vi "KLB or Jp2k3D Logging Control Module.vi"() -> ()   [LabVIEW 2012]
doc: "This vi is dynamically run at the start of an acquisition if logging type = jp2000 3D and acquisition mode = experiment. Stop by setting \"Stop?\" via vi server to True.\n\nThis vi continuously checks the JP2000 3D Images to log Buffer FG for \"Completed stack?\" = T; if found the completed stack is removed from the FG and passed to a PCITools VI to compress and then write the stack."
uses:
  PICTools/VIs/Error ring typedef.ctl
  JP2000 3D control/Jp2k 3D image file sets controller mode enum.ctl
  Error Handler/Non-announced error tracker modes enum.ctl
  subvi/KLB globals.vi
  Dynamic Parallel Logging/Parallel image logger globals.vi
  PICTools/VIs/PIC Tools.lvlib
  KLB.lvlib
panel:
  out "elapsed (ms)":u32
  out "# sets processed":i32
  out "last error=T":errorcluster
  out "Error Ring":T1 items=["ERR_NONE"=0, "ERR_EOF"=1, "ERR_SCAN_NON_EXIST"=2, "ERR_REQ_SCAN_NOT_IN_BUF"=3, "ERR_JUNK_BYTES_IN_HEADER"=4, "ERR_JUNK_BYTES_BEFORE_RESTART"=5, "ERR_RESTART_ATTEMPT_AFTER_BAD_DATA"=6, "ERR_TIFF_G34_PASTWIDTH_WARNING"=7, "ERR_MAXOUTPUTSIZE_TOO_SMALL"=8, "ERR_EXTRA_IMAGE_DATA"=9, "ERR_GIF_NO_MORE_PASSES"=10, "ERR_INSUFFICIENT_DATA_FOR_IPTC"=11, "ERR_WHILE_PARSING_IPTC"=12, "ERR_INTERNAL_WATCHDOG"=13, "ERR_NO_PIC_RESOURCE"=-1000, "ERR_BAD_DIB_SIZE"=-1001, "ERR_BAD_NUM_COLORS"=-1002, "ERR_BAD_NUM_GRAYS"=-1003, "ERR_CONFLICTING_REQUEST"=-1004, "ERR_BAD_SEEK"=-1005, "ERR_BAD_READ"=-1006, "ERR_OUT_OF_SPACE"=-1007, "ERR_BAD_DATA"=-1008, "ERR_BAD_IMAGE_TYPE"=-1009, "ERR_BAD_JPEG_DIB_HEADER"=-1010, "ERR_EXPAND_INTERNAL_ERR"=-1011, "ERR_SETUP_NOT_RUN"=-1012, "ERR_UNEXPECTED_EOF"=-1013, "ERR_BAD_WRITE"=-1014, "ERR_BAD_JPEG_COMPONENTS"=-1015, "ERR_UNIMPLEMENTED_FEATURE"=-1016, "ERR_BAD_SUBSAMPLING"=-1017, "ERR_TOO_MANY_INSTANCES"=-1018, "ERR_BAD_INSTANCE_ID"=-1019, "ERR_BAD_WIDTH_OR_HEIGHT"=-1020, "ERR_NOT_ENOUGH_BUFF_SPACE"=-1021, "ERR_BAD_DIB_DIM"=-1022, "ERR_BAD_QUANTIZATION_VALUE"=-1024, "ERR_OUT_OF_DATA"=-1025, "ERR_INCOMPATIBLE_JOIN"=-1026, "ERR_BAD_YUV_OUTPUT_TYPE"=-1027, "ERR_BAD_REGION_INFO"=-1028, "ERR_BAD_COLOR_TRANS_VAL"=-1029, "ERR_BAD_THUMBNAILLEN"=-1030, "ERR_BAD_THUMBNAILTOMAKE"=-1031, "ERR_THUMBNAIL_TOO_BIG"=-1032, "ERR_MISSING_THUMBNAIL"=-1033, "ERR_BAD_PIC2LIST"=-1034, "ERR_BAD_ENDIAN"=-1035, "ERR_CONFLICTING_PIC2LIST_PACKET"=-1036, "ERR_BAD_COLOR_TRANSFORM"=-1037, "ERR_UNSUPPORTED_NUM_COMPONENTS"=-1038, "ERR_STRIPSIZE_TOO_SMALL"=-1039, "ERR_STRIDE_TOO_SMALL"=-1040, "ERR_BAD_PLANAROFFSET"=-1041, "ERR_NOT_BASELINE"=-1101, "ERR_MARKER_ORDER"=-1102, "ERR_FRAME_HEADER"=-1103, "ERR_FILE_OR_FILE_READ"=-1104, "ERR_SCAN_HEADER"=-1105, "ERR_DNL_MARKER"=-1106, "ERR_NUM_LINES"=-1107, "ERR_RESTART"=-1108, "ERR_DC_RESTART"=-1109, "ERR_DECODE_DQ"=-1110, "ERR_DECODE"=-1111, "ERR_SKIP_DC"=-1112, "ERR_DECODE_THUMB"=-1113, "ERR_DECODE_MCU"=-1114, "ERR_SKIP_BLOCK"=-1115, "ERR_RENORM"=-1116, "ERR_AC_RESTART"=-1117, "ERR_DECODE_AC"=-1118, "ERR_DECODE_DC"=-1119, "ERR_BAD_BIT_COUNT"=-1201, "ERR_IMAGE_TOO_WIDE"=-1202, "ERR_MISSING_COLOR_MAP"=-1203, "ERR_BAD_REQUEST"=-1301, "ERR_EXPAND_BAD_SYNCH"=-1302, "ERR_BAD_ZOOM_DIB_HEADERS"=-1401, "ERR_BAD_DES_RECT"=-1402, "ERR_ZOOM_OUT_OF_RANGE"=-1403, "ERR_SRC_REC_TOO_BIG"=-1404, "ERR_DES_REC_TOO_BIG"=-1405, "ERR_BAD_SRC_REC_POS"=-1406, "ERR_BAD_DES_REC_POS"=-1407, "ERR_OUT_OF_ROOM"=-1408, "ERR_BAD_SRC_BITCOUNT"=-1409, "ERR_BAD_DES_BITCOUNT"=-1410, "ERR_COMPRESSED_IMAGE"=-1411, "ERR_BAD_SRC_PALETTE"=-1412, "ERR_BAD_DES_PALETTE"=-1413, "ERR_DES_DIB_TOO_SMALL"=-1414, "ERR_BAD_PIXELBITS"=-1415, "ERR_DIMENSIONS_DISAGREE"=-1416, "ERR_BAD_PIXELTYPES"=-1417, "ERR_BAD_PALETTE"=-1418, "ERR_OPERATION_NOT_INIT"=-1501, "ERR_OPERATION_ALREADY_INIT"=-1502, "ERR_WRONG_MODEL"=-1503, "ERR_UNKNOWN_REQUEST"=-1504, "ERR_UNKNOWN_RESPONSE"=-1505, "ERR_INVALID_OPERATION"=-1506, "ERR_INVALID_VERSION"=-1507, "ERR_GIVEN_BUFF_TOO_SMALL"=-1508, "ERR_APP_BUFF_NULL"=-1509, "ERR_COMMENT_BUFF_NULL"=-1510, "ERR_INVALID_USER_COLORS"=-1511, "ERR_CANT_CREATE_FULL_YUV_BUFF"=-1512, "ERR_NO_VALID_COLORS_AVAIL"=-1513, "ERR_GET_BUFF_INADEQUATE_PADDING"=-1514, "ERR_GET_BUFF_ERR"=-1515, "ERR_PUT_BUFF_ERR"=-1516, "ERR_NOT_8BIT_PRECISION"=-1517, "ERR_NOT_PROGRESSIVE"=-1518, "ERR_MISSING_KEY"=-1519, "ERR_INVALID_KEY"=-1520, "ERR_MAX_NUM_SCANS_EXCEEDED"=-1521, "ERR_UNSUPPORTED_JPEG_FORMAT"=-1522, "ERR_PUT_QUEUE_TOO_SMALL"=-1523, "ERR_TOO_MANY_RESTARTS"=-1524, "ERR_IMAGE_TOO_BIG"=-1525, "ERR_PUT_BUFF_TOO_SMALL"=-1526, "ERR_GET_QUEUE_TOO_SMALL"=-1527, "ERR_BAD_RESTART_INDEX"=-1528, "ERR_INVALID_LAYER"=-1529, "ERR_BAD_EOF"=-1530, "ERR_WRONG_PICL_VERSION"=-1531, "ERR_BAD_SCAN_PARMS"=-1532, "ERR_FULL_IMAGE_NOT_PRESENT"=-1533, "ERR_BAD_COMPRESSION_METHOD"=-1534, "ERR_BAD_COMPRESSION_ORDER"=-1535, "ERR_BAD_HUFFMAN_TABLE"=-1536, "ERR_BAD_QUANT_TABLE"=-1537, "ERR_NOT_LOSSLESS_JPEG"=-1538, "ERR_LJPEG_BAD_NUM_COMPONENTS"=-1539, "ERR_LJPEG_DOES_NOT_SUBSAMPLE"=-1540, "ERR_LJPEG_DOES_NOT_RESTART"=-1541, "ERR_LJPEG_BAD_DC_TABLE"=-1542, "ERR_LJPEG_TOO_MANY_HUFF_TABLES"=-1543, "ERR_LJPEG_MISSING_DIMENSIONS"=-1544, "ERR_LJPEG_BAD_PREDICTOR"=-1545, "ERR_LJPEG_BAD_POINT_TRANSFORM"=-1546, "ERR_QREVERSE"=-1547, "ERR_INTERNAL"=-1548, "ERR_BAD_PTUNING_VALUE"=-1549, "ERR_NOT_PIC2_FILE"=-1550, "ERR_BAD_PIC2_FORMAT"=-1551, "ERR_NOT_PCL2_FILE"=-1552, "ERR_BAD_PACKET_LENGTH"=-1553, "ERR_BAD_PCL2_PACKET"=-1554, "ERR_MISSING_PCL2_PACKET"=-1555, "ERR_BAD_PCL2_VERSION"=-1556, "ERR_BAD_MINOR_VERSION"=-1557, "ERR_TOO_MANY_BITS"=-1558, "ERR_LJPEG_INSUFFICIENT_SRC_ROOM"=-1559, "ERR_LJPEG_PUT_BUFF_TOO_SMALL"=-1560, "ERR_BITERR_MUST_BE_ZERO"=-1561, "ERR_LJPEG_RESTART_ERROR"=-1562, "ERR_LJPEG_BAD_ABE"=-1563, "ERR_LJPEG_BAD_AHT"=-1564, "ERR_IMPROPER_AHT_FOR_IMAGE"=-1565, "ERR_LJPEG_COLOR_NOT_24_BIT"=-1566, "ERR_LJPEG_BAD_MARKER_ORDER"=-1567, "ERR_LJPEG_R_G_OR_B_NOT_8_BITS"=-1568, "ERR_LJPEG_UNSUPPORTED_FILE_TYPE"=-1569, "ERR_BAD_REGION_TYPE"=-1570, "ERR_LJPEG_BAD_BIT_DEPTH"=-1571, "ERR_BAD_PARAMETER_VALUE"=-1572, "ERR_BAD_PRECISIONUCT"=-1573, "ERR_IPTC_TOO_LARGE_FOR_APPD"=-1574, "ERR_NOT_PROTECTED"=-1600, "ERR_BUFF_TOO_SMALL"=-1601, "ERR_WAVELET_INIT"=-1700, "ERR_WAVELET_COMPRESS"=-1701, "ERR_WAVELET_DECOMPRESS"=-1702, "ERR_BAD_IMAGENUMBER"=-1703, "ERR_CHUNKSIZE_TOO_SMALL"=-1704, "ERR_EXTRA_TABLE_OF_RECURSIVE"=-1705, "ERR_SHORT_TABLE_OF_RECURSIVE"=-1706, "ERR_MISSING_TABLE_OF_CLUSTERS"=-1707, "ERR_BAD_TRANSFORMFILTER"=-1708, "ERR_PNG_BAD_HEADER"=-1801, "ERR_PNG_BAD_SIGNATURE"=-1802, "ERR_PNG_MISSING_IHDR"=-1803, "ERR_PNG_BAD_IHDR"=-1804, "ERR_PNG_UNSUPPORTED_FEATURE"=-1805, "ERR_PNG_BAD_BIT_DEPTH"=-1806, "ERR_PNG_UNSUPPORTED_BIT_DEPTH"=-1807, "ERR_PNG_BAD_COLOR_TYPE"=-1808, "ERR_PNG_BAD_PLTE"=-1809, "ERR_PNG_MISSING_IDAT"=-1810, "ERR_PNG_BAD_CHUNK_TYPE"=-1811, "ERR_PNG_MISSING_PLTE"=-1812, "ERR_PNG_BAD_VERSION"=-1813, "ERR_PNG_INTERNAL_ERROR"=-1814, "ERR_PNG_STREAM_ERROR"=-1815, "ERR_PNG_INSUFFICIENT_DATA"=-1816, "ERR_PNG_BAD_CRC"=-1817, "ERR_PNG_BAD_CHUNK_ORDER"=-1818, "ERR_PNG_BAD_COMPRESSION"=-1819, "ERR_PNG_INVALID_FORMAT"=-1820, "ERR_INVALID_BACKGROUND"=-1821, "ERR_INVALID_TRANSPARENCY"=-1822, "ERR_WSQ_MISSING_MARKER"=-1901, "ERR_WSQ_MISSING_SOI"=-1902, "ERR_WSQ_MISSING_DIMENSIONS"=-1903, "ERR_WSQ_BAD_NUM_SUBBANDS"=-1904, "ERR_WSQ_BAD_HUFFMAN_TABLE_LEN"=-1905, "ERR_WSQ_MORE_THAN_8_HUFF_TABLES"=-1906, "ERR_WSQ_BAD_RESTART_HEADER"=-1907, "ERR_WSQ_BAD_FRAME_HEADER"=-1908, "ERR_WSQ_MISSING_SOB_MARKER"=-1909, "ERR_WSQ_UNEXPECTED_MARKER"=-1910, "ERR_WSQ_BAD_BLOCK_HEADER"=-1911, "ERR_WSQ_UNDEFINED_HUFFMAN_TABLE"=-1912, "ERR_WSQ_BAD_DTT_FILTERS"=-1913, "ERR_WSQ_MISSING_ANALYSIS_FILTER"=-1914, "ERR_WSQ_MISSING_SYNTHESIS_FILTER"=-1915, "ERR_WSQ_TOO_FEW_ECS_BLOCKS"=-1916, "ERR_WSQ_MISSING_FRAME_HEADER"=-1917, "ERR_WSQ_BAD_LOGFILE"=-1918, "ERR_WSQ_NO_ACTIVE_SUBBANDS"=-1919, "ERR_UNSUPPORTED_PLATFORM"=-1920, "ERR_NO_STATUS"=-2000, "ERR_USER_ABORTED"=-2001, "ERR_INTERNAL_INVALID_SREQUEST"=-2002, "ERR_HANDLE_NOT_FOUND"=-2003, "ERR_MEMORY_ALLOCATION_ERROR"=-2004, "ERR_FILE_OPEN_ERROR"=-2005, "ERR_DUPLICATE_ID"=-2006, "ERR_INVALID_HANDLE"=-2007, "ERR_LSEEK_ERROR"=-2008, "ERR_MORE"=-2009, "ERR_INTERNAL_POSTMESSAGE"=-2010, "ERR_LOCATE_SERVER_ERROR"=-2011, "ERR_INTERNAL_EXTRA_RESPONSE"=-2012, "ERR_INTERNAL_NOT_IN_PICLIST"=-2013, "ERR_INTERNAL_SHAREDINIT"=-2014, "ERR_INTERNAL_RESPONSE_SIZE"=-2015, "ERR_SERVER_RESPONSE_TIMEOUT"=-2016, "ERR_SERVER_MEMORY_ALLOCATION"=-2017, "ERR_SERVER_REQUEST_SIZE"=-2018, "ERR_SERVER_CLOSE"=-2019, "ERR_PUT_QUEUE_NULL"=-2020, "ERR_ALREADY_IN_PICLIST"=-2021, "ERR_INTERNAL_DELETE_RESPONSE"=-2022, "ERR_TOO_MANY_OPCODES_LOADED"=-2100, "ERR_OPCODE_DLL_NOT_FOUND"=-2101, "ERR_OPCODE_DLL_INVALID"=-2102, "ERR_OPCODE_INTERNAL_ERROR"=-2103, "ERR_OPCODE_INVALID_REG_CODE"=-2104, "ERR_OPCODE_UNSUPPORTED_PARMVER"=-2105, "ERR_LIB_NOT_INIT"=-2106, "ERR_CREATE_THREAD_ERROR"=-2107, "ERR_THREAD_EXITED"=-2108, "ERR_MEM_CHECK"=-2109, "ERR_CALLED_FROM_WRONG_THREAD"=-2110, "ERR_CALLED_FROM_WRONG_FIBER"=-2111, "ERR_DEFER_FROM_WRONG_THREAD"=-2112, "ERR_CREATE_MUTEX_ERROR"=-2113, "ERR_THREAD_ERROR"=-2114, "ERR_MUTEX_ERROR"=-2115, "ERR_EXTRASIZE_ZERO"=-2116, "ERR_DJVU_DECODE_ERR"=-2200, "ERR_DJVU_RENDER_ERR"=-2201, "ERR_DJVU_ENCODE_ERR"=-2202, "ERR_DJVU_MASK_ERR"=-2203, "ERR_DJVU_BADTEXTQUALITY"=-2204, "ERR_NULL_DEFERFN"=-2205, "ERR_DEFERFN_ABORT"=-2206, "ERR_DEFERFN_REQ_CONT"=-2207, "ERR_DEFERFN_16BIT_UNSUPPORTED"=-2208, "ERR_DEFERFN_NEST_PEGASUS"=-2209, "ERR_MODCA_BASE"=-2300, "ERR_MODCA_INVALID_SFI"=-2301, "ERR_MODCA_UNRECOGNIZED_ID"=-2302, "ERR_MODCA_EOD"=-2303, "ERR_IOCA_NOTBILEVEL"=-2304, "ERR_IOCA_EOD"=-2305, "ERR_IOCA_UNSUPPORTED"=-2306, "ERR_IOCA_INVALID"=-2307, "ERR_IOCA_BAD_WIDTH"=-2308, "ERR_CALS_BAD_HEADER"=-2309, "ERR_CALS_NO_WIDTH"=-2310, "ERR_CALS_UNSUPPORTED"=-2311, "ERR_CALS_BAD_RORIENT"=-2312, "ERR_BAD_WIDTHPAD"=-2313, "ERR_MODCA_INVALID_STRUCTURED_FIELD_IDENTIFIER"=-2314, "ERR_MODCA_UNRECOGNIZED_IDENTIFIER_CODE"=-2315, "ERR_MODCA_DATA_STREAM_STATE_VIOLATION"=-2316, "ERR_MODCA_UNRECOGNIZED_STRUCTURED_FIELD_OR_TRIPLET"=-2317, "ERR_MODCA_REQUIRED_STRUCTURED_FIELD_MISSING"=-2318, "ERR_MODCA_REQUIRED_PARAMETER_MISSING"=-2319, "ERR_MODCA_UNACCEPTABLE_PARAMETER_VALUE"=-2320, "ERR_MODCA_INCONSISTENT_PARAMETER_VALUES"=-2321, "ERR_MODCA_UNSUPPORTED"=-2322, "ERR_MODCA_UNABLE_TO_PARSE_PTOCA_FUNCTION"=-2323, "ERR_MODCA_WINDOWS_API_FAILED"=-2324, "ERR_MODCA_CANNOT_FIND_OVERLAY"=-2325, "ERR_MODCA_EXTERNAL_OVERLAY_IS_NULL"=-2326, "ERR_BAD_STATESTAMP"=-2400, "ERR_BAD_RCVRSTATE"=-2401, "ERR_BAD_ROI"=-2402, "ERR_RCVRSTATE_GET_MISMATCH"=-2403, "ERR_BAD_OUTPUTSIZE"=-2404, "ERR_BAD_CRC"=-2405, "ERR_IDP_VERSION_MISMATCH"=-2406, "ERR_BAD_SIGNATURE"=-2407, "ERR_NOT_JPEG_2000"=-2500, "ERR_BAD_MARKER"=-2501, "ERR_BAD_NUM_COMPONENTS"=-2503, "ERR_BAD_MARKER_ORDER"=-2504, "ERR_BAD_BIT_DEPTH"=-2509, "ERR_COLOR_NOT_24_BIT"=-2510, "ERR_BAD_NUM_TILES"=-2516, "ERR_COLOR_MAP_TO_RGB_NOT_8_BIT"=-2517, "ERR_BAD_PALETTE_INFO"=-2518, "ERR_BAD_COMPONENT_MAP_INFO"=-2519, "ERR_UNSUPPORTED_PIXEL_TYPE"=-2520, "ERR_OTHER_PARTITION_NOT_GRAY"=-2521, "ERR_TCT_WAVELET_TRANSFORMS_DIFFER"=-2522, "ERR_BAD_CHANNEL_TRANSFORMATION"=-2524, "ERR_BAD_TILE_DIMENSIONS"=-2526, "ERR_BAD_NUM_PARTITIONS"=-2527, "ERR_OUT_OF_SPACE_FOR_COMPONENT"=-2528, "ERR_INTERNAL_ERR"=-2530, "ERR_PUT_BUFFER_TOO_SMALL"=-2531, "ERR_QUEUE_MAY_NOT_BE_REVERSED"=-2532, "ERR_BAD_STRIDE"=-2534, "ERR_NULL_REGION"=-2535, "ERR_BAD_COMPRESSION_PROFILE"=-2536, "ERR_BAD_DECOMP_OR_SKIPPED_LEVELS"=-2537, "ERR_BAD_NUM_LAYERS"=-2538, "ERR_BAD_PROGRESSION_ORDER"=-2539, "ERR_BAD_TILE_COMP_TRANSFORM"=-2541, "ERR_BAD_WAVELET_TRANSFORM"=-2542, "ERR_BAD_IMAGE_WIDTH_OR_HEIGHT"=-2543, "ERR_BAD_TILE_WIDTH_OR_HEIGHT"=-2544, "ERR_BAD_TILE_OFFSET"=-2545, "ERR_BAD_TILE_ORIENTATION"=-2546, "ERR_COLORMAP_CAN_NOT_BE_SIGNED"=-2547, "ERR_BAD_CROP_PARAMETER"=-2548, "ERR_OFFSET_TOO_BIG"=-2549, "ERR_SIGNED_PIXELS_MAKING_BMP"=-2550, "ERR_BAD_BIT_DEPTH_MAKING_BMP"=-2551, "ERR_INSUFFICIENT_PARTITIONS"=-2552, "ERR_ONLY_2_TO_1_UPSAMPLING"=-2553, "ERR_SUBSAMPLED_CROP_UNSUPPORTED"=-2554, "ERR_UNSUPPORTED_COLOR_MAP_OPTION"=-2555, "ERR_CROP_AREA_EXCEEDS_IMAGE"=-2556, "ERR_PIC2LIST_HAS_DESCRIPTION"=-2557, "ERR_TOO_MANY_TILE_PARTS"=-2558, "ERR_BAD_PRECINCT_WIDTH_OR_HEIGHT"=-2559, "ERR_BAD_PSNR"=-2560, "ERR_BAD_RATE"=-2561, "ERR_BAD_LAYERRATE"=-2562, "ERR_BAD_COMPFILESIZE"=-2563, "ERR_UNSUPPORTED_BMP_IO"=-2564, "ERR_PARTITION_MISMATCH"=-2565, "ERR_UNSUPPORTED_SLICE_ENCODING"=-2566, "ERR_BAD_SLICE_OFFSET"=-2567, "ERR_UPDATEDTILES_NOT_ALLOWED"=-2568, "ERR_J2KLIB_WARNING"=-2569, "ERR_MODE_REQUIRES_SEEKING_ENABLED"=-2570, "ERR_BAD_SCAN_NUM"=-2601, "ERR_UNSUPPORTED_COMPONENT_DIMENSIONS"=-2602, "ERR_BAD_RESTART_INTERVAL"=-2605, "ERR_MISSING_DIMENSIONS"=-2608, "ERR_BAD_SYNCH_AT_EOS"=-2615, "ERR_MISSING_SOS"=-2616, "ERR_BAD_MAXVAL"=-2617, "ERR_BAD_RESET"=-2618, "ERR_BAD_NEARPARAM"=-2619, "ERR_BAD_ILVPARAM"=-2620, "ERR_BAD_PT"=-2621, "ERR_PTWITHMAP"=-2622, "ERR_BAD_MARKER_LENGTH"=-2623, "ERR_UNEXPECTED_UNKNOWN_LENGTH"=-2700, "ERR_UNSUPPORTED_UNPACKED_PIXELS"=-2701, "ERR_ENCODEMODE_LOSSY_TEXT_NOT_LOSSLESS"=-2702, "ERR_ENCODEMODE_LOSSY_HALFTONE_NOT_LOSSLESS"=-2703, "ERR_UNSUPPORTED_SEGMENT_REFERENCES"=-2704, "ERR_PCD_UNKNOWN_ERROR"=-3000, "ERR_PCD_BAD_FORMAT"=-3001, "ERR_PCD_BAD_PARAMETER"=-3002, "ERR_PCD_BAD_VERSION"=-3003, "ERR_PCD_READ_ERROR"=-3004, "ERR_PCD_CLOSE_ERROR"=-3005, "ERR_PCD_SEEK_ERROR"=-3006, "ERR_PCD_OPEN_ERROR"=-3007, "ERR_PCD_BAD_KEY"=-3008, "ERR_PCD_KEY_REQUIRED"=-3009, "ERR_PCD_ENCRYPTION_ERROR"=-3010, "ERR_PCD_NOT_INTERLEAVED"=-3011, "ERR_PCD_UNKNOWN_ATTRIBUTE"=-3012, "ERR_PCD_MEMORY_ERROR"=-3013, "ERR_PCD_SIZE_NOT_FOUND"=-3014, "ERR_OBJECT_INSTANCE_CORRUPT"=-3100, "ERR_BAD_X_VALUE"=-3101, "ERR_BAD_Y_VALUE"=-3102, "ERR_BAD_ARRAY_INDEX"=-3103, "ERR_BAD_RESOLUTION"=-3104, "ERR_BAD_DETECTION_QUALITY"=-3105, "ERR_BAD_SPECK_WIDTH"=-3106, "ERR_BAD_SPECK_HEIGHT"=-3107, "ERR_BAD_HORZ_LINE_MIN_LENGTH"=-3108, "ERR_BAD_HORZ_LINE_MAX_THICKNESS"=-3109, "ERR_BAD_HORZ_LINE_MIN_ASPECT_RATIO"=-3110, "ERR_BAD_HORZ_LINE_MAX_GAP"=-3111, "ERR_BAD_HORZ_LINE_MAX_CHAR_REPAIR_SIZE"=-3112, "ERR_BAD_HORZ_LINE_EDGE_CLEANING"=-3113, "ERR_BAD_VERT_LINE_MIN_LENGTH"=-3114, "ERR_BAD_VERT_LINE_MAX_THICKNESS"=-3115, "ERR_BAD_VERT_LINE_MIN_ASPECT_RATIO"=-3116, "ERR_BAD_VERT_LINE_MAX_GAP"=-3117, "ERR_BAD_VERT_LINE_MAX_CHAR_REPAIR_SIZE"=-3118, "ERR_BAD_VERT_LINE_EDGE_CLEANING"=-3119, "ERR_BAD_HORZ_ROTATION_ANGLE"=-3120, "ERR_BAD_VERT_ROTATION_ANGLE"=-3121, "ERR_BAD_SHEAR_ANGLE"=-3122, "ERR_BAD_AMOUNT_OF_EFFECT_LEFT"=-3123, "ERR_BAD_AMOUNT_OF_EFFECT_RIGHT"=-3124, "ERR_BAD_AMOUNT_OF_EFFECT_UP"=-3125, "ERR_BAD_AMOUNT_OF_EFFECT_DOWN"=-3126, "ERR_BAD_DIAGONAL_DIRECTION"=-3127, "ERR_BAD_RECT_WIDTH"=-3128, "ERR_BAD_RECT_HEIGHT"=-3129, "ERR_BAD_PAD_COLOR"=-3130, "ERR_BAD_MIN_DENSITY"=-3131, "ERR_BAD_MIN_PIXEL_COUNT"=-3132, "ERR_BAD_MAX_PIXEL_COUNT"=-3133, "ERR_BAD_HORIZONTAL_MAGNIFICATION"=-3134, "ERR_BAD_VERTICAL_MAGNIFICATION"=-3135, "ERR_BAD_MINIMUM_AREA_WIDTH"=-3136, "ERR_BAD_MINIMUM_AREA_HEIGHT"=-3137, "ERR_BAD_VERTICAL_SIZE_ADJUSTMENT"=-3138, "ERR_BAD_HORIZONTAL_SIZE_ADJUSTMENT"=-3139, "ERR_BAD_DENSITY"=-3140, "ERR_BAD_MAXIMUM_DOT_SIZE"=-3141, "ERR_BAD_VERIFICATION_HEIGHT"=-3142, "ERR_BAD_MINIMUM_BLACK_ON_EDGES"=-3143, "ERR_BAD_AMOUNT"=-3144, "ERR_IMAGE_TOO_SMALL"=-3145, "ERR_BAD_BORDER_SPECK_SIZE"=-3146, "ERR_BAD_PAGE_SPECK_SIZE"=-3147, "ERR_BAD_MINIMUM_PAGE_WIDTH"=-3148, "ERR_BAD_MAXIMUM_PAGE_WIDTH"=-3149, "ERR_BAD_MINIMUM_PAGE_HEIGHT"=-3150, "ERR_BAD_MAXIMUM_PAGE_HEIGHT"=-3151, "ERR_BAD_AMOUNT_TO_EXPAND_PAGE"=-3152, "ERR_BAD_HORZ_REG_RESULTANT_MARGIN"=-3153, "ERR_BAD_HORZ_REG_SKIP_DISTANCE"=-3154, "ERR_BAD_HORZ_REG_MIN_BACKGROUND"=-3155, "ERR_BAD_HORZ_REG_MIN_FOREGROUND"=-3156, "ERR_BAD_HORZ_REG_MIN_ACTIVITY"=-3157, "ERR_BAD_HORZ_REG_TO_LINE_MIN_LINE_LENGTH"=-3158, "ERR_BAD_HORZ_REG_TO_LINE_MAX_LINE_GAP"=-3159, "ERR_BAD_HORZ_REG_TO_LINE_MAX_LINE_THICKNESS"=-3160, "ERR_BAD_REG_ACTIVE"=-3161, "ERR_BAD_VERT_REG_RESULTANT_MARGIN"=-3163, "ERR_BAD_VERT_REG_SKIP_DISTANCE"=-3164, "ERR_BAD_VERT_REG_MIN_BACKGROUND"=-3165, "ERR_BAD_VERT_REG_MIN_FOREGROUND"=-3166, "ERR_BAD_VERT_REG_MIN_ACTIVITY"=-3167, "ERR_BAD_VERT_REG_TO_LINE_MIN_LINE_LENGTH"=-3168, "ERR_BAD_VERT_REG_TO_LINE_MAX_LINE_GAP"=-3169, "ERR_BAD_VERT_REG_TO_LINE_MAX_LINE_THICKNESS"=-3170, "ERR_BAD_COMB_LENGTH"=-3171, "ERR_BAD_COMB_HEIGHT"=-3172, "ERR_BAD_COMB_SPACING"=-3173, "ERR_BAD_COMB_H_LINE_THICKNESS"=-3174, "ERR_BAD_COMB_V_LINE_THICKNESS"=-3175, "ERR_BAD_COMB_MIN_CONFIDENCE"=-3176, "ERR_BAD_SENSITIVITY"=-3177, "ERR_BAD_MIN_SATURATION"=-3178, "ERR_BAD_MIN_SIZE"=-3179, "ERR_BAD_BOX_OVERLAP"=-3180, "ERR_BAD_COUNT"=-3181, "ERR_BAD_WHITE_BALANCE_METHOD"=-3200, "ERR_BAD_INTERPOLATION_METHOD"=-3201, "ERR_BAD_RED_FACTOR"=-3202, "ERR_BAD_BLUE_FACTOR"=-3203, "ERR_BAD_BRIGHTNESS_FACTOR"=-3204, "ERR_BAD_GAMMA"=-3205, "ERR_BAD_REGION_FLAGS"=-3206, "ERR_THUMBNAILBUFFER_NOT_NULL"=-3207, "ERR_REDEYE_RECT_LIST_TOO_SHORT"=-3300, "ERR_JPIP_BAD_REQUEST"=-3400, "ERR_JPIP_BAD_RESPONSE"=-3401, "ERR_UNKNOWN_ACTION"=-3402, "ERR_CHANNEL_NOT_OPEN"=-3403, "ERR_TOO_MANY_CHANNELS"=-3404, "ERR_TID_NOT_ALLOWED"=-3405, "ERR_TID_MISSING"=-3406, "ERR_CID_NOT_ALLOWED"=-3407, "ERR_CID_MISSING"=-3408, "ERR_UNSUPPORTED_TRANSPORT"=-3409, "ERR_BAD_JPIPREQUESTSTRING"=-3410, "ERR_BAD_JPIPRESPONSESTRING"=-3411, "ERR_BAD_TARGET"=-3412, "ERR_BAD_TARGETID"=-3413, "ERR_BAD_JPIPCHANNELID"=-3414, "ERR_BAD_JPIPCHANNELIDSCLOSE"=-3415, "ERR_BAD_MODEL"=-3416, "ERR_BAD_GRANTEDJPIPCHANNELID"=-3417, "ERR_BAD_GRANTEDJPIPCHANNELHOST"=-3418, "ERR_BAD_GRANTEDJPIPCHANNELPATH"=-3419, "ERR_BAD_EORMESSAGEBODY"=-3420, "ERR_STATELESS_SECOND_REQUEST"=-3421, "ERR_NOT_DEFAULT_MEDIATYPE"=-3422, "ERR_UNSUPPORTED_MEDIATYPE"=-3423, "ERR_NOT_ALLOWED_TRANSPORT"=-3424, "ERR_BAD_TPMODEL"=-3425, "ERR_UNSUPPORTED_JPX_FORMAT"=-3500, "ERR_BAD_JPEG2000PROFILE"=-3501, "ERR_BAD_JPEG2000FILEFORMAT"=-3502, "ERR_BAD_TILECOMPFLAGS"=-3503, "ERR_BAD_THUMBNAIL"=-3504, "ERR_TOO_MANY_DISCARD_LAYERS"=-3505, "ERR_BAD_RESOLUTIONBOX_VALUE"=-3506, "ERR_MISSING_ICC_PROFILE_DATA"=-3507, "ERR_EXIFIFD_CONTEXT"=-3600, "ERR_GPSINFOIFD_CONTEXT"=-3601, "ERR_INTEROPERABILITYIFD_CONTEXT"=-3602, "ERR_LIBRARY_ERROR"=-3603, "ERR_BAD_PIXTYPE"=-3604, "ERR_UNSUPPORTED_PIXELFORMAT"=-3605, "ERR_BAD_OVERLAP"=-3606, "ERR_BAD_TRIMMED_FLEXBITS"=-3607, "ERR_BAD_SUBBANDS"=-3608, "ERR_BAD_ALPHA_CHANNEL_FORMAT"=-3609, "ERR_IMAGE_DATA_MUST_BE_UNCOMPRESSED"=-3610, "ERR_SUBSAMPLING_DISALLOWED_FOR_PIXTYPE"=-3611, "ERR_BAD_REORIENTATION"=-3612, "ERR_UNSUPPORTED_INPUT_IMAGE"=-3613, "JWBASE"=-7000, "ERR_UNEXPECTED_RESPONSE"=-7002, "ERR_OUT_OF_MEMORY"=-7003, "ERR_UNSUPPORTED_FILE_TYPE"=-7004, "ERR_BAD_STRUCTURE_PARAMETER"=-7005, "ERR_INVALID_HEADER_INFO"=-7006, "ERR_BAD_RLE_DATA"=-7007, "ERR_RLE_DELTA_UNSUPPORTED"=-7008, "ERR_BAD_BMP_TYPE"=-7009, "ERR_NULL_POINTER"=-7010, "ERR_BAD_TGA_TYPE"=-7011, "ERR_UNSUPPORTED_BIT_DEPTH"=-7012, "ERR_UNSUPPORTED_RLE_MODE"=-7013, "ERR_BAD_PCX_PALETTE"=-7014, "ERR_NOT_BMP_FILE"=-7015, "ERR_NOT_TARGA_FILE"=-7016, "ERR_NOT_PCX_FILE"=-7017, "ERR_NOT_GIF_FILE"=-7018, "ERR_BAD_GIF_SEPARATOR"=-7019, "ERR_DIFFERENT_GIF_FORMAT"=-7020, "ERR_GIF_DECODE_ERROR_1"=-7021, "ERR_GIF_DECODE_ERROR_2"=-7022, "ERR_GIF_DECODE_ERROR_3"=-7023, "ERR_GIF_DECODE_ERROR_4"=-7024, "ERR_GIF_DECODE_ERROR_5"=-7025, "ERR_GIF_DECODE_ERROR_6"=-7026, "ERR_BAD_GIF_EXTENSION_BLOCK"=-7027, "ERR_NOT_TIFF_FILE"=-7028, "ERR_INVALID_TIFF_IFD_COUNT"=-7029, "ERR_INVALID_TIFF_TAG"=-7030, "ERR_TIFF_NO_JPEG"=-7031, "ERR_TIFF_NO_CCITT"=-7032, "ERR_TIFF_NO_DIFFERENCING"=-7033, "ERR_TIFF_NO_TILES"=-7034, "ERR_TIFF_NO_CMYK"=-7035, "ERR_TIFF_NO_YCbCr"=-7036, "ERR_TIFF_BAD_PHOTOMETRIC"=-7037, "ERR_TIFF_UNSUPPORTED_COMPRESSION"=-7038, "ERR_TIFF_NO_STRIP_INFO"=-7039, "ERR_TIFF_NEED_COLORMAP"=-7040, "ERR_TIFF_PALETTE_WRONG_SIZE"=-7041, "ERR_TIFF_BAD_STRIPOFFSETS_TYPE"=-7042, "ERR_TIFF_NO_WIDTH_OR_LENGTH"=-7043, "ERR_TIFF_TOO_FEW_STRIPS"=-7044, "ERR_TIFF_TAG_COUNT_SHOULD_BE_1"=-7045, "ERR_TIFF_UNEXPECTED_TYPE"=-7046, "ERR_TIFF_BAD_ARRAY_TYPE"=-7047, "ERR_TIFF_BAD_ARRAY_COUNT"=-7048, "ERR_TIFF_BAD_BITS_PER_SAMPLE"=-7049, "ERR_UNKNOWN_UTILITY_FUNCTION"=-7050, "ERR_BAD_OUTPUT_BPP"=-7051, "ERR_BAD_INPUT_PALETTE"=-7052, "ERR_INVALID_NUMBER_OF_OUTPUT_COLORS"=-7053, "ERR_BAD_INPUT_PIXEL_DEPTH"=-7054, "ERR_DIB_MUST_BE_UNCOMPRESSED"=-7055, "ERR_MISSING_PALETTE"=-7056, "ERR_INVALID_STRUCTURE_SIZE"=-7057, "ERR_BAD_PROGRESSIVE_MODE"=-7058, "ERR_NOT_YET_IMPLEMENTED"=-7059, "ERR_BAD_NUMBER_OF_PLANES"=-7060, "ERR_INVALID_TARGA_BPP"=-7061, "ERR_UNSUPPORTED_INPUT_PIXEL_DEPTH"=-7062, "ERR_TIFF_LOGIC_ERROR_1"=-7063, "ERR_TIFF_LOGIC_ERROR_2"=-7064, "ERR_TIFF_OUTPUT_WIDTH_0"=-7065, "ERR_UTL_HISTOGRAM_IS_NULL"=-7066, "ERR_UTL_COLORMAP_IS_NULL"=-7067, "ERR_TOO_MANY_COLORS_IN_COLORMAP"=-7068, "ERR_DIB_MUST_BE_24BPP"=-7069, "ERR_INVALID_HISTOGRAM_SIZE"=-7070, "ERR_UNSUPPORTED_TGA_ATT_BITS"=-7071, "ERR_UNIMPLEMENTED_SUBCODE"=-7072, "ERR_TIFF_UNSUPPORTED_ORIENTATION"=-7073, "ERR_TIFF_NO_SAMPLEFORMAT"=-7074, "ERR_TIFF_UNSUPPORTED_DATATYPE"=-7075, "ERR_SUB8_PTR3_NULL"=-7076, "ERR_PALETTE_SIZE"=-7077, "ERR_COLOR_COUNT_MISMATCH"=-7078, "ERR_BAD_DIB_DEPTH"=-7079, "ERR_UTL_NO_EXTERNAL_PALETTE"=-7080, "ERR_SUB8_LOGIC_ERROR_1"=-7081, "ERR_OUTPUT_QUEUE_TOO_SMALL"=-7082, "ERR_SUBCODE_INTERNAL_1"=-7083, "ERR_SUBCODE_INTERNAL_2"=-7084, "ERR_SUBCODE_INTERNAL_3"=-7085, "ERR_SUBCODE_INTERNAL_4"=-7086, "ERR_SUBCODE_INTERNAL_5"=-7087, "ERR_PCD_NOT_VALID_COMPRESSION"=-7088, "ERR_PCD_NO_NAME"=-7089, "ERR_PCD_BAD_RESOLUTION"=-7090, "ERR_TIFF_G34_1"=-7091, "ERR_TIFF_G34_2"=-7092, "ERR_TIFF_G34_3"=-7093, "ERR_TIFF_G34_4"=-7094, "ERR_TIFF_G34_5"=-7095, "ERR_TIFF_G34_6"=-7096, "ERR_TIFF_G34_7"=-7097, "ERR_TIFF_G34_8"=-7098, "ERR_TIFF_G3_DECODE_1"=-7099, "ERR_TIFF_G3_DECODE_2"=-7100, "ERR_TIFF_G3_DECODE_3"=-7101, "ERR_TIFF_G3_DECODE_4"=-7102, "ERR_TIFF_LZW_DECODE_1"=-7103, "ERR_TIFF_BAD_PREDICTOR"=-7104, "ERR_TIFF_UNSUPPORTED_PLANARCONFIGURATION"=-7105, "ERR_TIFF_UNSUPPORTED_SAMPLES_PER_PIXEL"=-7106, "ERR_QUEUE_ERROR"=-7107, "ERR_TIFF_BAD_FILLORDER"=-7108, "ERR_TIFF_G34_RAWWIDTH0"=-7109, "ERR_TIFF_G34_INVALIDEOL"=-7110, "ERR_TIFF_G34_PASTWIDTH"=-7111, "ERR_TIFF_G34_PREMATUREEOS"=-7112, "ERR_TIFF_G34_FIRSTLINE2D"=-7113, "ERR_TIFF_G34_EXTENSIONCODE"=-7114, "ERR_TIFF_G34_INVALIDCODE"=-7115, "ERR_TIFF_G34_SEQUENCE"=-7116, "ERR_TIFF_G34_G32DMISSINGEOL"=-7117, "ERR_INVALID_BISIZE"=-7118, "ERR_INVALID_CMYK_PARAMETERS"=-7119, "ERR_PUTQ_UNEXPECTED_EOF"=-7120, "ERR_PUTQ_BAD_READ"=-7121, "ERR_PUTQ_GET_BUFF_ERR"=-7122, "ERR_TIFF_INVALID_MULTI_ENDIAN"=-7123, "ERR_TIFF_NO_LOSSLESS_JPEG"=-7124, "ERR_TIFF_JPEG_STRIPS"=-7125, "ERR_TIFF_INVALID_PAGE"=-7126, "ERR_TIFF_DUPLICATE_TAG"=-7127, "ERR_THRESHOLD_EXCEEDED"=-7128, "ERR_BAD_THRESHOLD"=-7129, "ERR_BAD_OFFSET"=-7130, "ERR_BAD_DCX_IMAGE"=-7131, "ERR_OUT_OF_ROOM_IN_DCX_FILE"=-7132, "ERR_BAD_CONTRASTFIXEDPOINT"=-7133, "ERR_ALPHA_UNSUPPORTED_FOR_INPUT"=-7134, "ERR_SAVE_ALPHA_REQUIRES_ALPHA_INPUT"=-7135, "ERR_ALPHA_UNSUPPORTED_FOR_OUTPUT"=-7136, "ERR_MASKBUFFERSIZE_TOO_SMALL"=-7137, "ERR_NO_TILE_OFFSETS"=-7138, "ERR_UNSUPPORTED_TILE_WIDTH"=-7139, "ERR_DAMAGED_FILE"=-7200, "ERR_INVALID_DICT"=-7201, "ERR_INVALID_TYPE"=-7202, "ERR_INVALID_HEADER"=-7203, "ERR_MISSING_RESOURCES"=-7204, "ERR_BLANK_PAGE"=-7205, "ERR_NO_IMAGE_FOUND"=-7206, "ERR_INVALID_IMAGE_BPP"=-7207, "ERR_INVALID_IMAGE_HEIGHT"=-7208, "ERR_INVALID_IMAGE_WIDTH"=-7209, "ERR_INVALID_STREAM_LENGTH"=-7210, "ERR_INVALID_PAGE_NUMBER"=-7211, "ERR_INVALID_DICT_KEY"=-7212, "ERR_DAMAGED_XREF_SECTION"=-7213, "ERR_MAX_ARRAY_SIZE_REACHED"=-7214, "ERR_MAX_DICT_SIZE_REACHED"=-7215, "ERR_MAX_STR_LENGTH_REACHED"=-7216, "ERR_MAX_NAME_LENGTH_REACHED"=-7217, "ERR_INVALID_STREAM"=-7218, "ERR_MULT_DECODE_PARMS_NOT_SUPPORTED"=-7219, "ERR_MULT_FILTERS_NOT_SUPPORTED"=-7220, "ERR_UNEXPECTED_NULL_OBJECT"=-7221, "ERR_MULT_CONTENT_STREAMS_NOT_SUPPORTED"=-7222, "ERR_ENCODED_STREAMS_NOT_SUPPORTED"=-7223, "ERR_COLOR_SPACE_NOT_SUPPORTED"=-7224, "ERR_NO_IMAGE_SCALE_TRANSFORM_FOUND"=-7225, "ERR_XREF_OBJ_FOR_TRAILER_NOT_SUPPORTED"=-7226, "ERR_LAYOUT_DOES_NOT_EXIST"=-7300, "ERR_TRUNCATE64"=-7900, "ERR_J2KLIB_OFFSET"=-8000, "ERR_UNEXPECTED_ERROR"=-9000]
  out "Compression Ratio":dbl=2.0
  in  "Stop?":bool
  out "error out":errorcluster
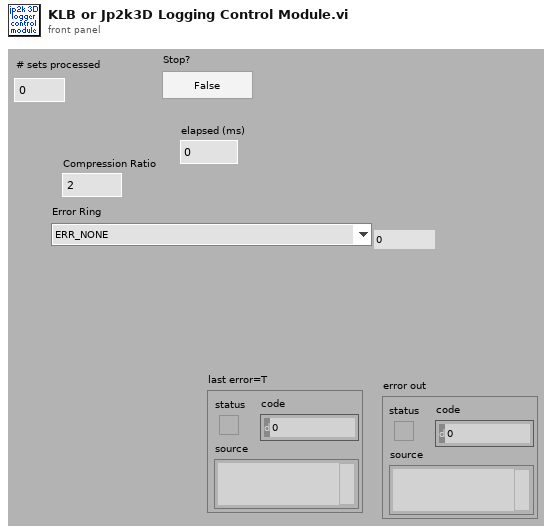
[diagram p1: front panel]
types:
  T1 = typedef "PIC Tools.lvlib/Error ring typedef.ctl" = i32
  T2 = typedef "Jp2k 3D image file sets controller mode enum.ctl" = enum16{"Initialize", "Read registers", "Add Image", "Remove element", "Mark all done 1 camera"}
  T3 = typedef "Non-announced error tracker modes enum.ctl" = enum16{"Reset", "Add error", "Read registers"}
  T4 = typedef "Jp2k file SET cluster.ctl" = cluster{"Path":path, "Camera index":i32, "[Buffer #]":i32[], "Completed?":bool}
  T5 = typedef "IMAQ Image.ctl" = refnum<image>
  T6 = typedef "KLB.lvlib/KLB Settings Cluster.ctl" = cluster{"Logical Cores":T7, "pixelSize (um)":sgl[], "blockSize":u32[], "compressionType":T8, "metadata":string}
  T7 = typedef "KLB.lvlib/KLB # of CPUs enum.ctl" = enum16{"CPU 25%", "CPU 50%", "CPU 75%", "CPU All but 1", "1", "4", "8", "16"}
  T8 = typedef "KLB.lvlib/KLB compression type enum.ctl" = enum8{"Uncompressed", "BZip2"}
  T9 = typedef "PIC Tools.lvlib/Compression options cluster.ctl" = cluster{"Number of Threads":i32, "Lossless compression":bool, "3D compression":bool, "Compression Ratio":dbl}
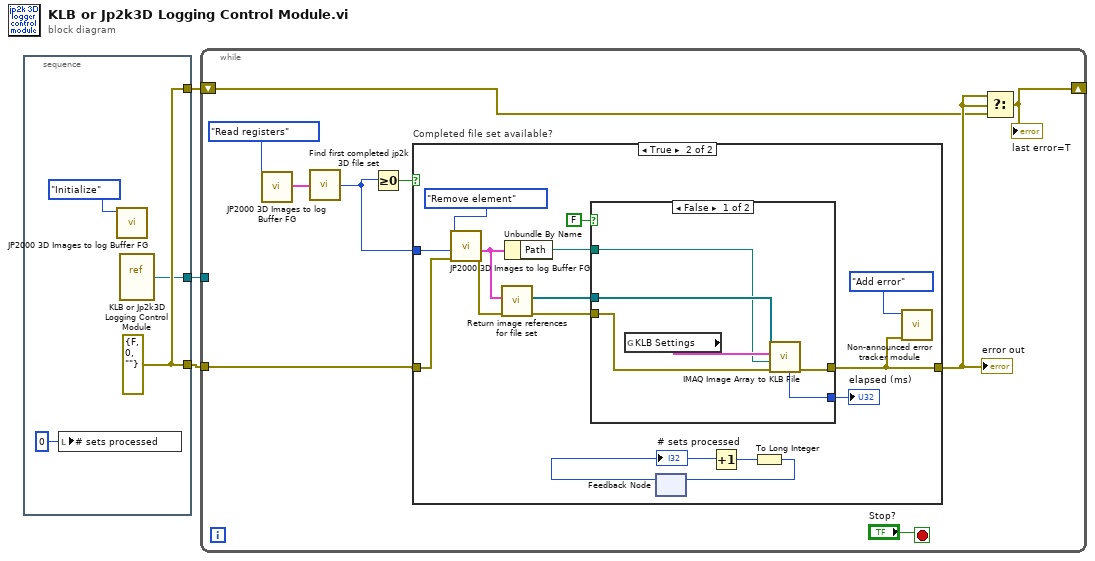
[diagram p0: block diagram]
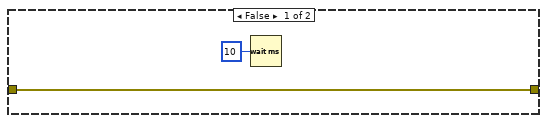
[diagram p2: hidden frame]
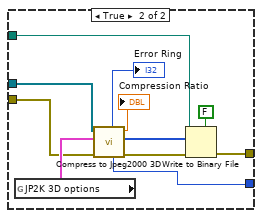
[diagram p3: hidden frame]
diagram:
  n1 = stacked-sequence {
    tunnel: [w6] -> w3
    tunnel: [w6] -> w2
    tunnel: [w5] -> w1
    frame #0 {
      w6 = errorcluster {"status"=FALSE, "code"=0, "source"=""} ("error out")
      n2 = local write "# sets processed"(0 ("# sets processed")) -> ()
      n3 = call "JP2000 3D Images to log Buffer FG.vi"("Mode"=Jp2k_3D_image_file_sets_controller_mode_enum."Initialize") -> ()  [unwired: 8 in, 3 out]
      n4 = vi-ref "KLB or Jp2k3D Logging Control Module.vi"() -> (w5:refnum<vi>)
    }
  }
  n5 = while {
    tunnel: w3 -> [w11]
    shift-right: [w8] -> _
    shift-left: w2 -> [w9]
    tunnel: w1 -> [_]
    stop <- "Stop?" stop-if-true
    n6 = call "JP2000 3D Images to log Buffer FG.vi"("Mode"=Jp2k_3D_image_file_sets_controller_mode_enum."Read registers") -> ("[File sets]"=w13:T4[])  [unwired: 8 in, 2 out]
    n7 = call "Find first completed jp2k 3D file set.vi"("[File sets]"=w13) -> ("1st Completed index"=w12:i32)  [unwired: 4 in]
    n8 = Greater Or Equal To 0?(x=w12) -> (x >= 0?=w15:bool)
    n9 = case "Completed file set available?" shown="True" w15 {
      tunnel: [w18 w21] -> w10
      tunnel: w11 -> [w18 w27]
      tunnel: w12 -> [_ w33]
      frame False {
        n10 = Wait (ms)(milliseconds to wait=u32 10) -> ()  [unwired: 1 out]
      }
      frame True {
        n11 = call "JP2000 3D Images to log Buffer FG.vi"("error in (no error)"=w27, "Index"=w33, "Mode"=Jp2k_3D_image_file_sets_controller_mode_enum."Remove element") -> ("error out"=w26:errorcluster, "Removed element"=w30:T4)  [unwired: 6 in, 1 out]
        n12 = call "Return image references for file set.vi"("error in (no error)"=w26, "Removed element"=w30) -> ("error out"=w29:errorcluster, "Images"=w28:T5[])  [unwired: 8 in]
        n13 = Unbundle By Name(w30) -> ("Path"=w32:path)
        n14 = case shown="False" FALSE {
          tunnel: w32 -> [w36 w46]
          tunnel: w29 -> [w35 w43]
          tunnel: w28 -> [w38 w42]
          tunnel: [w39 w41] -> w21
          tunnel: [w34 w40] -> w19
          frame False {
            n15 = global read "KLB globals.vi" "KLB Settings"() -> (w37:T6)
            n16 = call "IMAQ Image Array to KLB File.vi"("error in (no error)"=w35, "path"=w36, "KLB Settings"=w37, "Images to Compress"=w38) -> ("error out"=w39:errorcluster, "elapsed (ms)"=w34:u32)  [unwired: 6 in]
          }
          frame True {
            n17 = global read "Parallel image logger globals.vi" "JP2K 3D options"() -> (w50:T9)
            n18 = call "Compress to Jpeg2000 3D.vi"("error in"=w43, "Compression options"=w50, "Images to Compress"=w42) -> ("error out"=w48:errorcluster, "OutputBuffer"=w47:u8[], "Compression Ratio achieved"=→"Compression Ratio":dbl, "elapsed (ms)"=w40:u32, "Error Ring"=→"Error Ring":T1)  [unwired: 3 in, 1 out]
            n19 = Write to Binary File(file (use dialog)=w46, data=w47, error in=w48, 5:FALSE ("prepend array or string size? (T)")) -> (error out=w41:errorcluster)  [unwired: 2 in, 2 out]
          }
        }
        "elapsed (ms)" <- w19
        n20 = feedback #1() -> (w24:i32)  [unwired: 1 in]
        "# sets processed" <- w24
        n21 = Increment(x=w24) -> (x+1=w25:i32)
        n22 = To Long Integer(number=w25) -> (32bit integer=w23:i32)
        n23 = feedback-in #1(w23) -> ()
        n24 = call "Non-announced error tracker module.vi"("error in"=w21, "Mode"=Non-announced_error_tracker_modes_enum."Add error") -> ()  [unwired: 7 in, 3 out]
      }
    }
    "error out" <- w10
    n25 = Select(t=w10, s=w10, f=w9) -> (s? t:f=w8:errorcluster)
    "last error=T" <- w8
  }
